vi "c_ctre_phoenix6_platform_write_schema_value.vi"(0 "String 2":string, 1 "String 4":string, 2 "Numeric 2":u16, 3 "Numeric 4":u8, 4 "Numeric 5":u32, 5 "Numeric 6":dbl) -> (20 "Numeric":i32, 21 "String":string, 22 "String 3":string, 23 "Numeric 3":u8)   [LabVIEW 2025]
uses:
  <vilib>/Rock Robotics/WPI/ThirdParty/Phoenix-LabVIEW/Controls/DriverLib.ctl
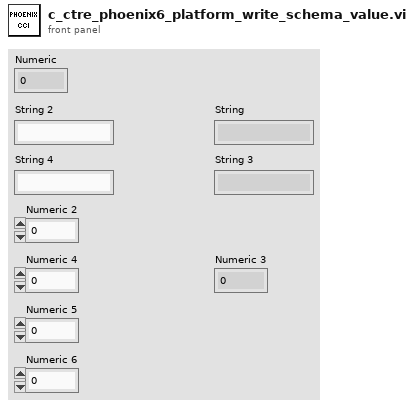
[diagram p1: front panel]
types:
  T1 = typedef "DriverLib.ctl" = path
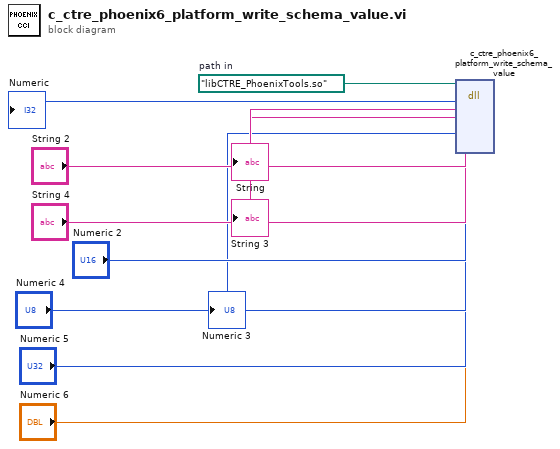
[diagram p0: block diagram]
diagram:
  w11 = T1 path "libCTRE_PhoenixTools.so"  # path in
  n1 = dll-call lib="?" fn="c_ctre_phoenix6_platform_write_schema_value"(path in=w11, "String 2", "String 4", "Numeric 2", "Numeric 4", "Numeric 5", "Numeric 6") -> (→"Numeric":i32, →"String":string, →"String 3":string, →"Numeric 3":u8)  [unwired: 5 in, 2 out]
